vi "Read from Inline Execution Units.vi"(8 "error in (no error)":errorcluster, 11 "RTStateVariables in":T1 {"Inline Execution Units"."Outgoing Data References"."Data Reference" format="%.0x"; "Inline Execution Units"."Incoming Data References" format="%.0x"}) -> (0 "error out":errorcluster, 3 "RTStateVariables out":T1 {"Inline Execution Units"."Outgoing Data References"."Data Reference" format="%.0x"; "Inline Execution Units"."Incoming Data References" format="%.0x"})   [LabVIEW 2020, in "AIM ARINC 429 Engine.lvlib" / "Custom Device.lvlib"]
uses:
  Custom Device.lvlib
  <vilib>/NI VeriStand/Custom Device API/Custom Device API.lvlib
  Interfaces/Execution Unit/Execution Unit.lvclass
  <vilib>/NI/NIVS Inline Async API/_VS Inline Async API/VS Inline Async API/VS Inline Async API.lvclass
  RTStateVariables.ctl
  <vilib>/NI VeriStand/Custom Device API/Data Reference.ctl
  <vilib>/NI VeriStand/Custom Device API/Block Data Reference.ctl
  Inline Execution Unit Runtime Information.ctl
  Asynchronous Execution Unit Runtime Information.ctl
  Interfaces/Shared Resources/Shared Resources.lvclass
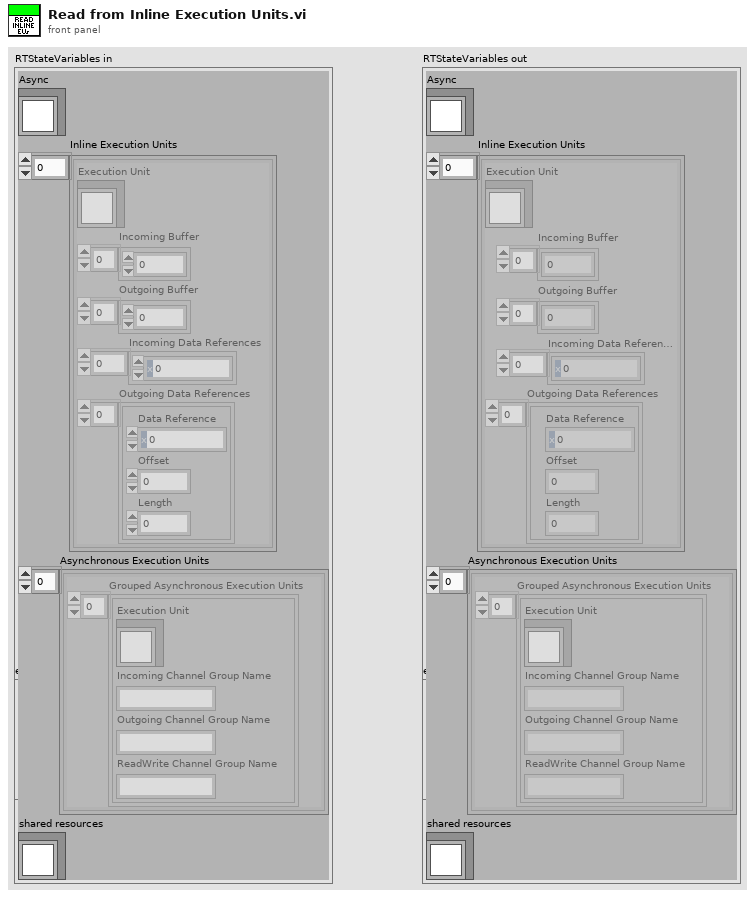
[diagram p1: front panel]
types:
  T1 = typedef "AIM ARINC 429 Engine.lvlib/Custom Device.lvlib/RTStateVariables.ctl" = cluster{"Async":refnum<class "VS Inline Async API.lvclass">, "Inline Execution Units":T2[], "Asynchronous Execution Units":cluster{"Grouped Asynchronous Execution Units":T5[]}[], "shared resources":refnum<class "Shared Resources.lvclass">}
  T2 = typedef "AIM ARINC 429 Engine.lvlib/Custom Device.lvlib/Inline Execution Unit Runtime Information.ctl" = cluster{"Execution Unit":refnum<class "Execution Unit.lvclass">, "Incoming Buffer":dbl[], "Outgoing Buffer":dbl[], "Incoming Data References":T3[], "Outgoing Data References":T4[]}
  T3 = typedef "Custom Device API.lvlib/Data Reference.ctl" = i32
  T4 = typedef "Custom Device API.lvlib/Block Data Reference.ctl" = cluster{"Data Reference":T3, "Offset":u64, "Length":u64}
  T5 = typedef "AIM ARINC 429 Engine.lvlib/Custom Device.lvlib/Asynchronous Execution Unit Runtime Information.ctl" = cluster{"Execution Unit":refnum<class "Execution Unit.lvclass">, "Incoming Channel Group Name":string, "Outgoing Channel Group Name":string, "ReadWrite Channel Group Name":string}
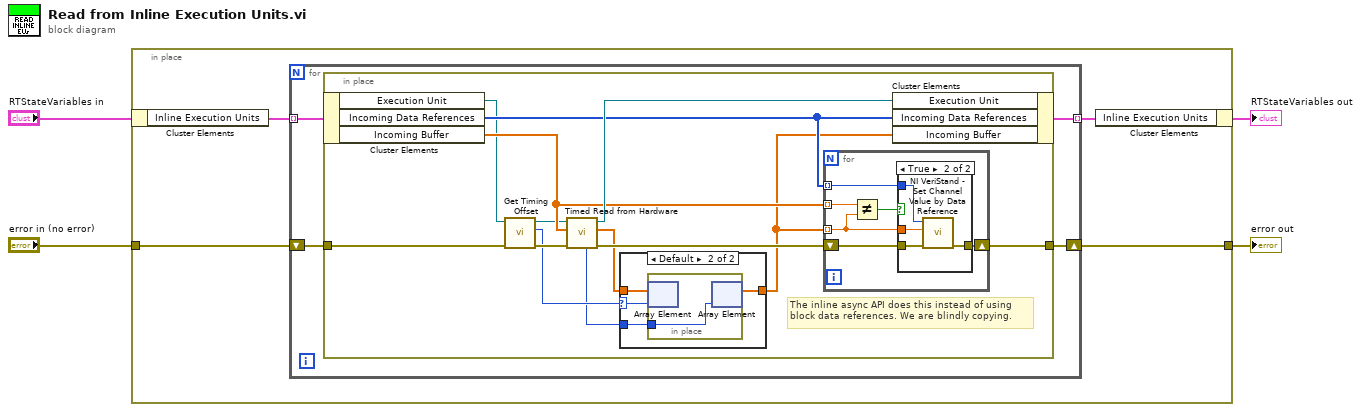
[diagram p0: block diagram]
diagram:
  n1 = in-place {
    in-place-border: [w8] -> w4
    in-place-border: "error in (no error)" -> [w7]
    n2 = in-place-cluster #1("RTStateVariables in") -> ("Inline Execution Units"=w6:T2[])
    n3 = for {
      tunnel: [w10] -> w5 mode=indexing
      tunnel: w6 -> [w9] mode=indexing
      shift-right: [w12] -> w8
      shift-left: w7 -> [w11]
      n4 = in-place {
        in-place-border: w11 -> [w19]
        in-place-border: [w23] -> w12
        # "The inline async API does this instead of using\nblock data references. We are blindly copying."
        n5 = in-place-cluster #2(w9) -> ("Execution Unit"=w20:refnum<class "Execution Unit.lvclass">, "Incoming Data References"=w22:T3[], "Incoming Buffer"=w21:dbl[])
        n6 = call-dynamic "Get Timing Offset.vi"("error in (no error)"=w19, "Execution Unit in"=w20) -> ("error out"=w18:errorcluster, "Timing Channel Offset"=w16:i64, "Execution Unit out"=w17:refnum<class "Execution Unit.lvclass">)  [unwired: 7 in]
        n7 = call "Timed Read from Hardware.vi"("error in"=w18, "Values in"=w21, "Execution Unit in"=w17) -> ("error out"=w24:errorcluster, "Values out"=w15:dbl[], "Execution Unit out"=w25:refnum<class "Execution Unit.lvclass">, "Execution Duration (us)"=w13:u32)  [unwired: 5 in]
        n8 = case shown="Default" w16 {
          selector: w16 -> [_ w39]
          tunnel: w15 -> [w37 w41]
          tunnel: [w37 w40] -> w14
          tunnel: w13 -> [_ w38]
          frame ..-1 {
          }
          frame Default {
            n9 = in-place {
              in-place-border: w38 -> [w42]
              n10 = in-place-array #3(w41, w39) -> ()  [unwired: 1 out]
              n11 = in-place-array #3(w42) -> (w40:dbl[])  [unwired: 1 out]
            }
          }
        }
        n12 = for {
          tunnel: w21 -> [w28] mode=indexing
          tunnel: w14 -> [w27] mode=indexing
          shift-right: [w29] -> w23
          shift-left: w24 -> [w30]
          tunnel: w22 -> [w26] mode=indexing
          n13 = Not Equal?(x=w28, y=w27) -> (x != y?=w31:bool)
          n14 = case shown="True" w31 {
            tunnel: w30 -> [w32 w36]
            tunnel: [w32 w35] -> w29
            tunnel: w27 -> [_ w34]
            tunnel: w26 -> [_ w33]
            frame False {
            }
            frame True {
              n15 = call <vilib>:"NI VeriStand - Set Channel Value by Data Reference.vi"("error in (no error)"=w36, "Value"=w34, "Data Reference in"=w33) -> ("error out"=w35:errorcluster)  [unwired: 8 in]
            }
          }
        }
        n16 = in-place-cluster #2("Execution Unit"=w25, "Incoming Data References"=w22, "Incoming Buffer"=w14) -> (w10:T2)
      }
    }
    n17 = in-place-cluster #1("Inline Execution Units"=w5) -> (→"RTStateVariables out":T1)
  }
  "error out" <- w4
